vi "ZPL Config Transient Mode.vi"(6 "Settle (1 mS)":u32=1, 7 "Step & Counter":cluster{"Step":u16, "Counter (Default:1)":dbl}={"Step"=0, "Counter (Default:1)"=1.0} {"Counter (Default:1)" min=1.0 max=9999.0 step=1.0; "Step" items=["ONCE", "AUTO"]}, 8 "error":errorcluster, 9 "Values":T1, 10 "MODE":cluster{"Mode":u16, "Transient Mode (None)":u16} caption="Cluster 1" {"Transient Mode (None)" items=["NONE", "FIX", "LIST", "WAVE"]; "Mode" items=["VOLTAGE", "CURRENT"]}, 11 "VISA":refnum<visa-resource-name>="0") -> (0 "error out":errorcluster={"status"=FALSE, "code"=-1073807343, "source"=""}, 3 "VISA out":refnum<visa-resource-name>="0")   [LabVIEW 2015]
doc: "This VI sets the advance waveform. There are four modes \nNONE - is regular operation. \nFIX - In this mode of output control, each triggered output voltage or current value is explicitly specified by a triggered-level command (for example, VOLT:TRIG 20 or CURR:TRIG 1.55). The trigger then causes the output to change to this pending triggered level.\nLIST - This mode occurs when the VOLT:MODE LIST or CURR:MODE LIST command is programmed. In this mode of output operation, the triggered output voltage or current levels are specified within a list and the trigger controls the sequencing through the values in the list.\nWAVE -This mode occurs when the VOLT:MODE WAVE or CURR:MODE WAVE command is programmed. In this mode of output operation, the triggered output voltage or current levels and rise and fall slope are specified within a list and the trigger controls the sequencing through the values in the list."
panel:
  out "String":string
  # "Lambda ZPLUS \n Serial Port\n  DC Power Supplies"
  # "Config Transient mode\n( NONE, FIX, LIST, WAVE)"
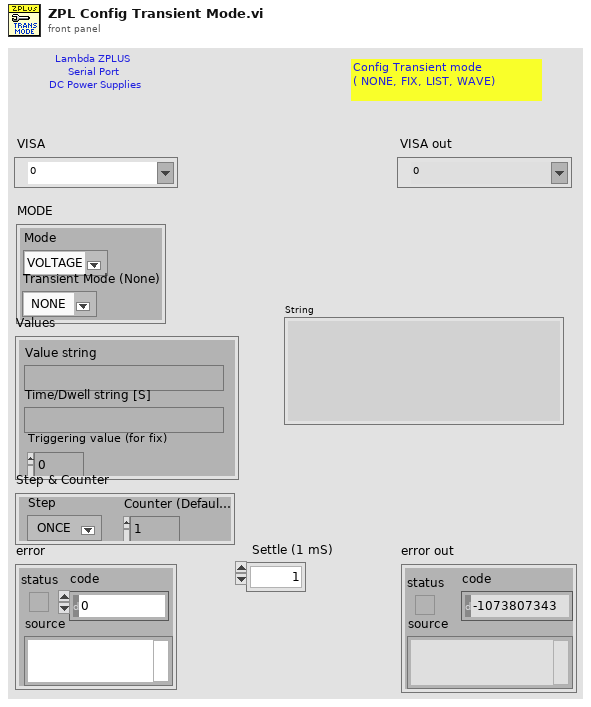
[diagram p1: front panel]
types:
  T1 = cluster{"Value string":string, "Time/Dwell string [S]":string, "Triggering value (for fix)":dbl}
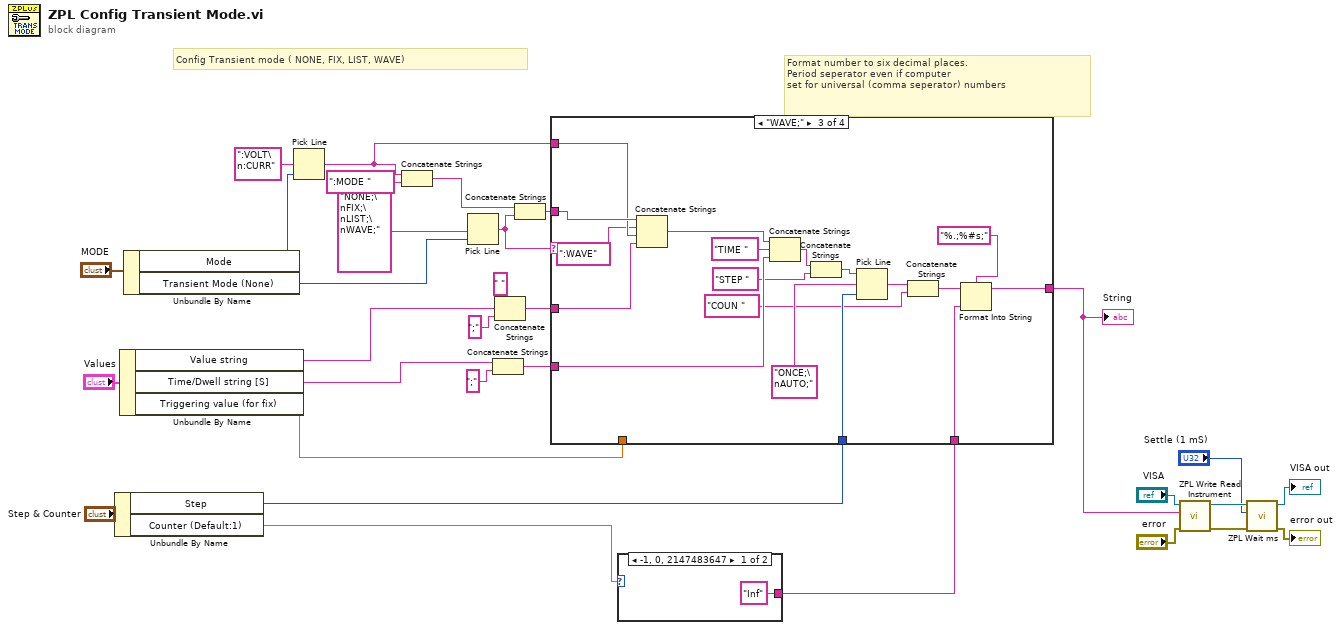
[diagram p0: block diagram]
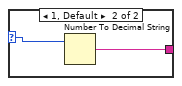
[diagram p2: hidden frame]
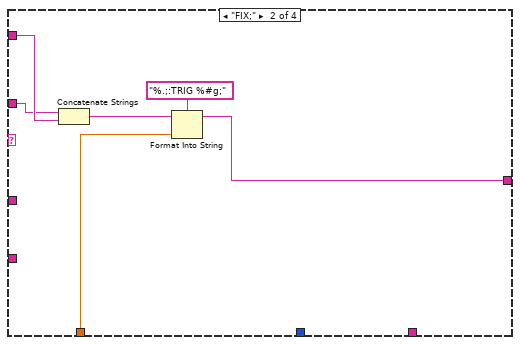
[diagram p4: hidden frame]
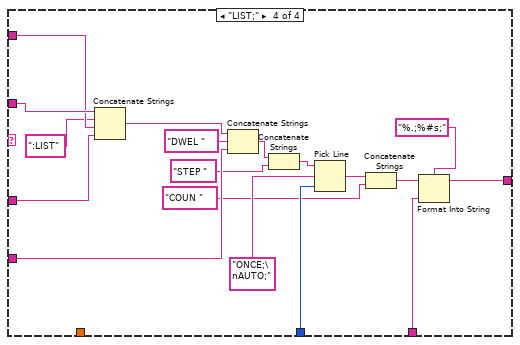
[diagram p5: hidden frame]
diagram:
  # "Format number to six decimal places.\nPeriod seperator even if computer \nset for universal (comma seperator) numbers"
  # "Config Transient mode ( NONE, FIX, LIST, WAVE)"
  n1 = Unbundle By Name("Step & Counter") -> ("Step"=w3:u16, "Counter (Default:1)"=w2:dbl)
  n2 = Unbundle By Name("Values") -> ("Value string"=w5:string, "Time/Dwell string [S]"=w6:string, "Triggering value (for fix)"=w7:dbl)
  n3 = Unbundle By Name("MODE") -> ("Mode"=w10:u16, "Transient Mode (None)"=w9:u16)
  n4 = Pick Line(multi-line string=":VOLT\n:CURR" ("format string"), line index=w10) -> (output string=w21:string)  [unwired: 1 in]
  n5 = Concatenate Strings(w21, ":MODE " ("string")) -> (w18:string)
  n6 = Pick Line(multi-line string="NONE;\nFIX;\nLIST;\nWAVE;", line index=w9) -> (output string=w19:string)  [unwired: 1 in]
  n7 = Concatenate Strings(w6, ";" ("string")) -> (w12:string)
  n8 = Concatenate Strings(" " ("string"), w5, ";" ("string")) -> (w15:string)
  n9 = Concatenate Strings(w18, w19) -> (w17:string)
  n10 = case shown="-1, 0, 2147483647" w2 {
    selector: w2 -> [_ w34]
    tunnel: ["Inf" w33] -> w1
    frame -1, 0, 2147483647 {
    }
    frame 1, Default {
      n11 = Number To Decimal String(number=w34) -> (decimal integer string=w33:string)  [unwired: 1 in]
    }
  }
  n12 = case shown="\"WAVE;\"" w19 {
    tunnel: w21 -> [_ w40 w58 w76]
    tunnel: [w35 w38 w42 w60] -> w20
    tunnel: w17 -> [w35 w37 w59 w77]
    tunnel: w15 -> [_ _ w57 w75]
    tunnel: w12 -> [_ _ w54 w72]
    tunnel: w7 -> [_ w36 _ _]
    tunnel: w3 -> [_ _ w52 w70]
    tunnel: w1 -> [_ _ w43 w61]
    frame "False", Default {
    }
    frame "FIX;" {
      n13 = Concatenate Strings(w37, w40) -> (w39:string)
      n14 = Format Into String(format string="%.;:TRIG %#g;", initial string=w39, w36) -> (resulting string=w38:string)  [unwired: 1 in, 1 out]
    }
    frame "WAVE;" {
      n15 = Concatenate Strings(w59, ":WAVE" ("string"), w58, w57) -> (w56:string)
      n16 = Concatenate Strings(w56, "TIME " ("string"), w54) -> (w49:string)
      n17 = Concatenate Strings(w49, "STEP " ("string")) -> (w50:string)
      n18 = Pick Line(string ("")=w50, multi-line string="ONCE;\nAUTO;" ("format string"), line index=w52) -> (output string=w47:string)
      n19 = Concatenate Strings(w47, "COUN " ("string")) -> (w44:string)
      n20 = Format Into String(format string="%.;%#s;", initial string=w44, w43) -> (resulting string=w42:string)  [unwired: 1 in, 1 out]
    }
    frame "LIST;" {
      n21 = Concatenate Strings(w77, ":LIST" ("string"), w76, w75) -> (w74:string)
      n22 = Concatenate Strings(w74, "DWEL " ("string"), w72) -> (w67:string)
      n23 = Concatenate Strings(w67, "STEP " ("string")) -> (w68:string)
      n24 = Pick Line(string ("")=w68, multi-line string="ONCE;\nAUTO;" ("format string"), line index=w70) -> (output string=w65:string)
      n25 = Concatenate Strings(w65, "COUN " ("string")) -> (w62:string)
      n26 = Format Into String(format string="%.;%#s;", initial string=w62, w61) -> (resulting string=w60:string)  [unwired: 1 in, 1 out]
    }
  }
  "String" <- w20
  n27 = call "ZPL Write Read Instrument.vi"("error in"="error", "Write Command/Query SCPI"=w20, "VISA"="VISA") -> ("error out"=w28:errorcluster, "VISA  out"=w29:refnum<visa-resource-name>)  [unwired: 6 in, 1 out]
  n28 = call "ZPL Wait ms.vi"("error"=w28, "Delay (1 mS)"="Settle (1 mS)", "VISA"=w29) -> ("error out"=→"error out":errorcluster, "VISA out"=→"VISA out":refnum<visa-resource-name>)  [unwired: 7 in]
